vi "Filter Outliers.vi"(11 "Targets":T1(array[cluster])) -> (3 "Targets Out":T1(array[cluster]))   [LabVIEW 2011]
panel:
  in  "Max Error":dbl=10.0
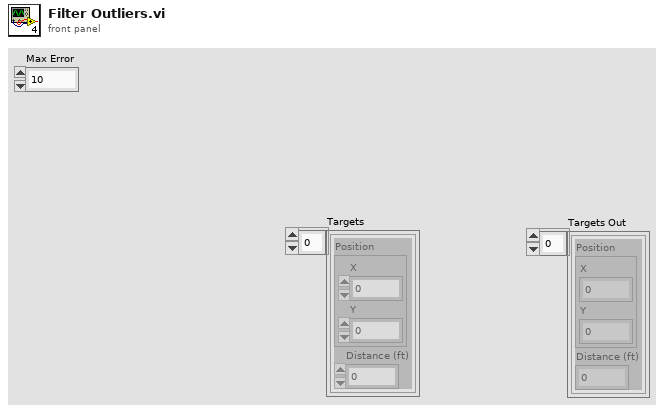
[diagram p1: front panel]
types:
  T1 = cluster{"Position":cluster{"X":dbl, "Y":dbl}, "Distance (ft)":dbl}[]
  T2 = cluster{"Position":cluster{"X":dbl, "Y":dbl}, "Distance (ft)":dbl}
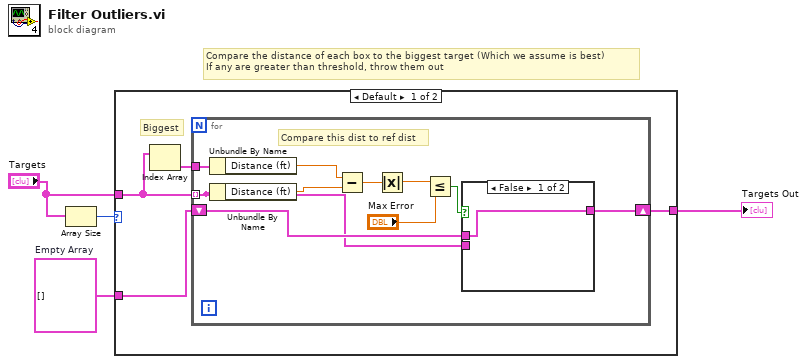
[diagram p0: block diagram]
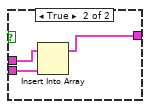
[diagram p2: hidden frame]
diagram:
  w1 = T1 []  # Empty Array
  # "Compare the distance of each box to the biggest target (Which we assume is best)\nIf any are greater than threshold, throw them out"
  n1 = Array Size(array="Targets") -> (size(s)=w4:i32)
  n2 = case shown="Default" w4 {
    tunnel: "Targets" -> [w6 w23]
    tunnel: [w8 w23] -> w2
    tunnel: w1 -> [w5 _]
    frame Default {
      # "Biggest"
      n3 = Index Array(array=w6) -> (element=w7:T2)  [unwired: 1 in]
      n4 = for {
        shift-right: [w11] -> w8
        shift-left: w5 -> [w12]
        tunnel: w7 -> [w18]
        tunnel: w6 -> [w10] mode=indexing
        # "Compare this dist to ref dist"
        n5 = Unbundle By Name(w18) -> ("Distance (ft)"=w17:dbl)
        n6 = Unbundle By Name(w10) -> ("Distance (ft)"=w16:dbl)
        n7 = Subtract(x=w17, y=w16) -> (x-y=w15:dbl)
        n8 = Absolute Value(x=w15) -> (abs(x)=w14:dbl)
        n9 = Less Or Equal?(x=w14, y="Max Error") -> (x <= y?=w9:bool)
        n10 = case shown="False" w9 {
          tunnel: w12 -> [w19 w22]
          tunnel: [w19 w21] -> w11
          tunnel: w10 -> [_ w20]
          frame False {
          }
          frame True {
            n11 = Insert Into Array(array=w22, new element=w20) -> (w21:T1)  [unwired: 1 in]
          }
        }
      }
    }
    frame 0 {
    }
  }
  "Targets Out" <- w2
